vi "vacuum_Q.vi"(7 "cmd":enum16{"create", "write", "read", "close"}(ring), 8 "error in":errorcluster, 11 "data":enum16{"config", "run", "pause", "stop"}(ring)) -> (0 "error out":errorcluster, 3 "queue out":refnum<queue>)   [LabVIEW 2013]
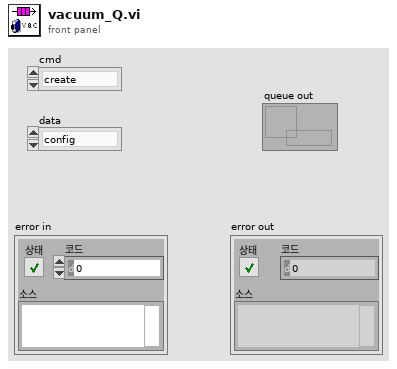
[diagram p1: front panel]
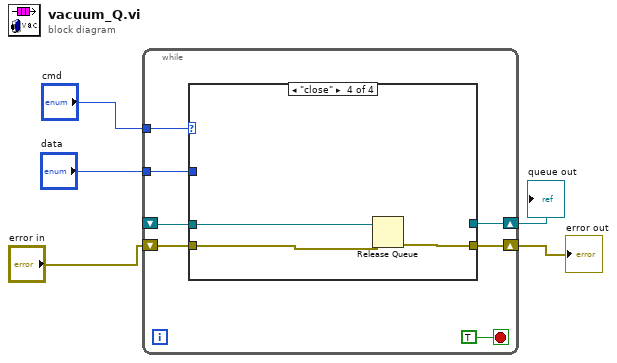
[diagram p0: block diagram]
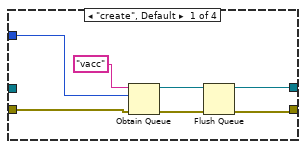
[diagram p2: hidden frame]
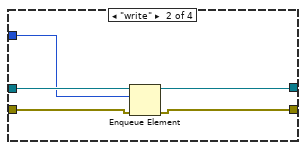
[diagram p3: hidden frame]
diagram:
  n1 = while {
    tunnel: "cmd" -> [w11]
    shift-right: [w9] -> w3
    shift-left: "error in" -> [w10]
    shift-right: [w8] -> w1
    shift-left: _ -> [w7]
    tunnel: "data" -> [w6]
    stop <- TRUE stop-if-true
    n2 = case shown="\"close\"" w11 {
      tunnel: w10 -> [w19 w24 w25 w28]
      tunnel: [w13 w23 w25 w29] -> w9
      tunnel: [w14 w22 w26 _] -> w8
      tunnel: w7 -> [_ w21 w26 w27]
      tunnel: w6 -> [w18 w20 _ _]
      frame "create", Default {
        n3 = Obtain Queue(name (unnamed)="vacc" ("이름(이름없음)"), element data type=w18, error in (no error)=w19) -> (queue out=w15:refnum<queue>, error out=w16:errorcluster)  [unwired: 2 in, 1 out]
        n4 = Flush Queue(queue=w15, error in (no error)=w16) -> (queue out=w14:refnum<queue>, error out=w13:errorcluster)  [unwired: 1 out]
      }
      frame "write" {
        n5 = Enqueue Element(queue=w21, element=w20, error in (no error)=w24) -> (queue out=w22:refnum<queue>, error out=w23:errorcluster)  [unwired: 1 in, 1 out]
      }
      frame "read" {
      }
      frame "close" {
        n6 = Release Queue(queue=w27, error in (no error)=w28) -> (error out=w29:errorcluster)  [unwired: 1 in, 2 out]
      }
    }
  }
  "error out" <- w3
  "queue out" <- w1
